vi "IsFreeField.vi"(7 "SnakesOnly?":bool, 8 "error in (no error)":errorcluster, 10 "Coordinate":cluster{"x":i16, "y":i16}, 11 "SnakeGame in":refnum<class "SnakeGame.lvclass">) -> (0 "error out":errorcluster, 2 "Free?":bool, 3 "SnakeGame out":refnum<class "SnakeGame.lvclass">)   [LabVIEW 2019, in "RT_Game.lvlib" / "SnakeGame.lvclass"]
uses:
  SnakeGame.lvclass
  SnakeGame.lvclass/SnakeGame.ctl
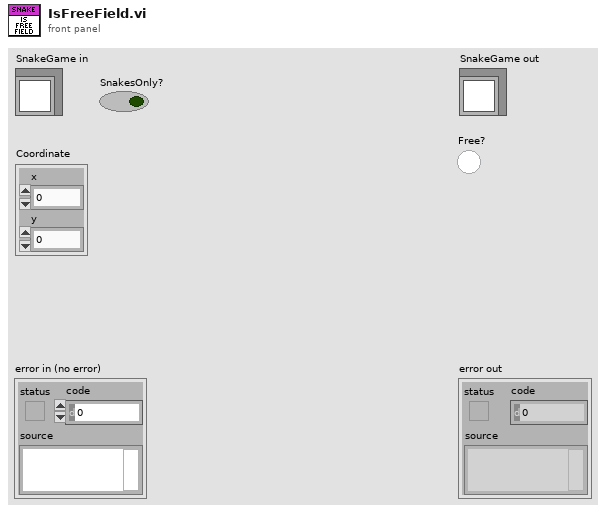
[diagram p1: front panel]
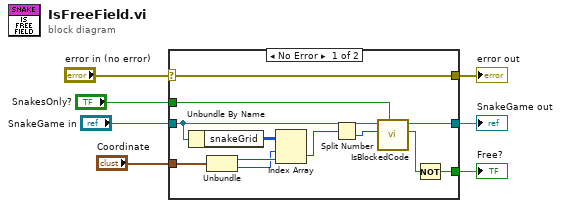
[diagram p0: block diagram]
diagram:
  n1 = case shown="No Error" "error in (no error)" {
    selector: "error in (no error)" -> [w19 w21]
    tunnel: [w19 w21] -> w6
    tunnel: [w13 w20] -> w4
    tunnel: "SnakeGame in" -> [w18 w20]
    tunnel: "Coordinate" -> [w16 _]
    tunnel: [w10 _] -> w2
    tunnel: "SnakesOnly?" -> [w8 _]
    frame No Error {
      n2 = Unbundle By Name(w18) -> ("snakeGrid"=w17:u32[][])
      n3 = Unbundle(w16) -> ("x"=w15:i16, "y"=w14:i16)
      n4 = Index Array(array=w17, index (row)=w14, index (col)=w15) -> (element=w12:u32)
      n5 = Split Number(x=w12) -> (lo(x)=w9:u16)  [unwired: 1 out]
      n6 = call "IsBlockedCode.vi"("SnakesOnly?"=w8, "Code"=w9, "SnakeGame in"=w18) -> ("Blocked?"=w11:bool, "SnakeGame out"=w13:refnum<class "SnakeGame.lvclass">)  [unwired: 7 in]
      n7 = Not(x=w11) -> (.not. x?=w10:bool)
    }
    frame Error {
    }
  }
  "error out" <- w6
  "SnakeGame out" <- w4
  "Free?" <- w2
